vi "getAllChannels.vi"(8 "error in (no error)":errorcluster, 11 "deviceDataBase in":refnum<class "deviceDataBase.lvclass">) -> (0 "error out":errorcluster, 2 "ChannelArray.lvclass":refnum<class "ChannelArray.lvclass">, 3 "deviceDataBase out":refnum<class "deviceDataBase.lvclass">)   [LabVIEW 2009, in "Tools.lvlib" / "DatabaseHelpers.lvlib" / "deviceDataBase.lvclass"]
uses:
  deviceDataBase.lvclass
  Database Objects/ChannelArray/ChannelArray.lvclass
  deviceDataBase.lvclass/deviceDataBase.ctl
  Database Objects/DeviceArray/DeviceArray.lvclass
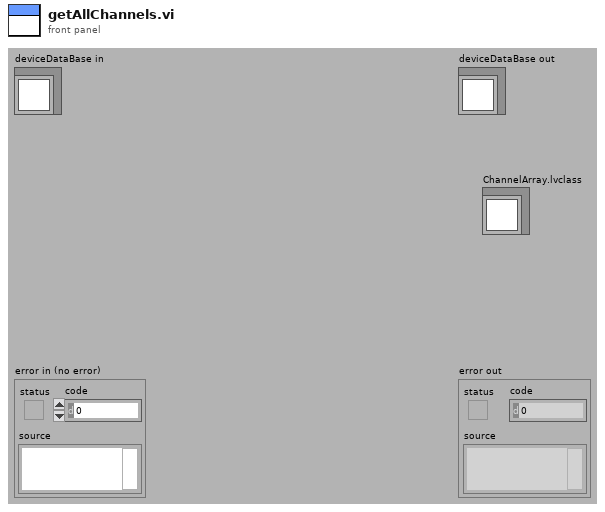
[diagram p1: front panel]
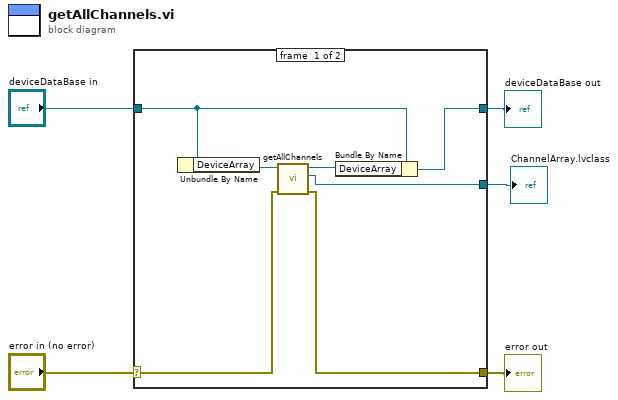
[diagram p0: block diagram]
diagram:
  n1 = case shown="No Error" "error in (no error)" {
    selector: "error in (no error)" -> [w10 w14]
    tunnel: [w9 w14] -> w4
    tunnel: [w6 w13] -> w2
    tunnel: "deviceDataBase in" -> [w7 w13]
    tunnel: [w11 _] -> w1
    frame #0 {
      n2 = Unbundle By Name(w7) -> ("DeviceArray"=w12:refnum<class "DeviceArray.lvclass">)
      n3 = call "getAllChannels.vi"("error in (no error)"=w10, "DeviceArray in"=w12) -> ("error out"=w9:errorcluster, "ChannelArray.lvclass"=w11:refnum<class "ChannelArray.lvclass">, "DeviceArray out"=w8:refnum<class "DeviceArray.lvclass">)  [unwired: 7 in]
      n4 = Bundle By Name(cluster=w7, "DeviceArray"=w8) -> (w6:refnum<class "deviceDataBase.lvclass">)
    }
    frame #1 {
    }
  }
  "error out" <- w4
  "deviceDataBase out" <- w2
  "ChannelArray.lvclass" <- w1
